vi "VCI_CloseDevice.vi"(2 "error in (no error)":errorcluster, 3 "DevIndex":u32, 4 "DevType":u32) -> (0 "error out":errorcluster, 1 "CloseDevice_Success?":u32)   [LabVIEW 2014]
uses:
  ControlCAN.dll
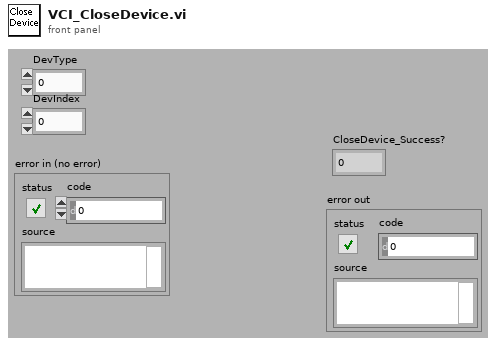
[diagram p1: front panel]
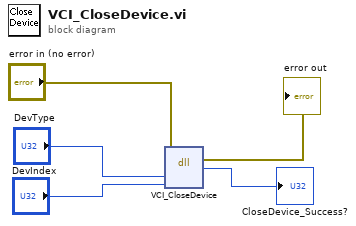
[diagram p0: block diagram]
diagram:
  n1 = dll-call lib="PTH22abs D\tDocuments\tCan总线canControlCAN.dll" fn="VCI_CloseDevice"(error in="error in (no error)", "DevType"="DevType", "DevIndex"="DevIndex") -> (error out=→"error out":errorcluster, "CloseDevice_Success?"=→"CloseDevice_Success?":u32)  [unwired: 4 in, 1 out]
